vi "PyGet3.vi"(0 "Attribute":string) -> (1 "Error":bool, 2 "Reply":string)   [LabVIEW 2014]
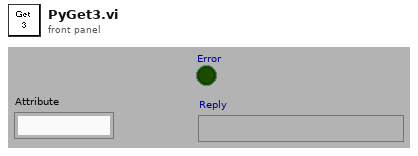
[diagram p1: front panel]
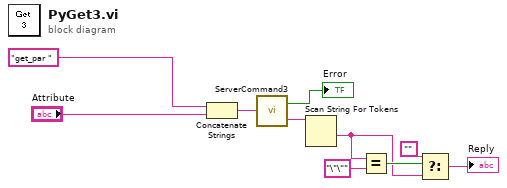
[diagram p0: block diagram]
diagram:
  n1 = Concatenate Strings("get_par " ("string"), "Attribute") -> (w10:string)
  n2 = call "ServerCommand3.vi"("Command"=w10) -> ("Error"=→"Error":bool, "Reply"=w8:string)
  n3 = Scan String For Tokens(9:w8) -> (1:w4:string)  [unwired: 5 in, 3 out]
  n4 = Equal?(x=w4, y="\"\"") -> (x = y?=w5:bool)
  n5 = Select(t="", s=w5, f=w4) -> (s? t:f=→"Reply":string)
